vi "Untitled 3 (SubVI).vi"(11 "Numeric in":dbl) -> (3 "Numeric out":dbl)   [LabVIEW 2018]
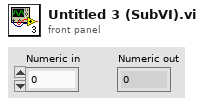
[diagram p1: front panel]
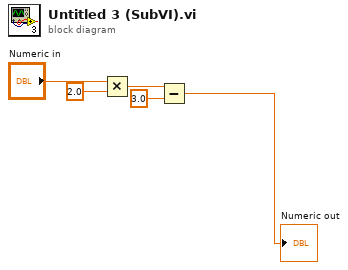
[diagram p0: block diagram]
diagram:
  n1 = Multiply(x="Numeric in", y=2.0) -> (x*y=w3:dbl)
  n2 = Subtract(x=w3, y=3.0) -> (x-y=→"Numeric out":dbl)
